vi "Load.vi"(8 "error in (no error)":errorcluster, 11 "reference in":refnum<class "DUT_Handler_Simple.lvclass">) -> (0 "error out":errorcluster, 1 "OK":bool, 3 "reference in":refnum<class "DUT_Handler_Simple.lvclass">)   [LabVIEW 2022 SP3, in "DUT_Handler_Simple.lvlib" / "DUT_Handler_Simple.lvclass"]
uses:
  DUT_Handler_Simple.lvclass
  Components/DUT_Handler_Base.lvlibp/Action.ctl
  Components/DUT_Handler_Base.lvlibp/EventData.ctl
  Components/DUT_Handler_Base.lvlibp/DUT_Handler_Base.lvclass
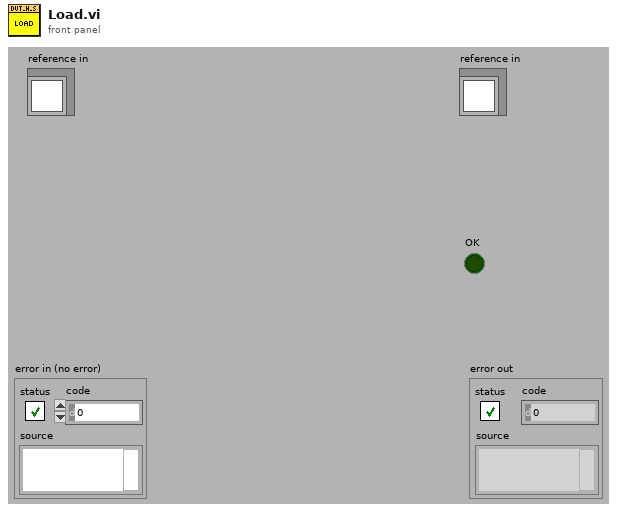
[diagram p1: front panel]
types:
  T1 = typedef "DUT_Handler_Base.lvlibp/DUT_Handler_Base.lvclass/EventData.ctl" = cluster{"Action":enum16{"Load", "Cancel", "MoveIn", "MoveOut", "Abort", "Msg", "Enabled", "Disabled", "Fault", "Shutdown"}, "SN":string, "BN":string, "DUT__ID":u32, "Message":string, "From":string, "To":string}
  T2 = typedef "DUT_Handler_Base.lvlibp/DUT_Handler_Base.lvclass/Action.ctl" = enum16{"Load", "Cancel", "MoveIn", "MoveOut", "Abort", "Msg", "Enabled", "Disabled", "Fault", "Shutdown"}
  T3 = typedef "DUT_Handler_Simple.lvlib/DUT_Handler_Simple.lvclass/ObjectAttributes.ctl" = cluster{"Config":T4, "event_data":T1, "Enabled":bool, "Barcode_Reader":refnum<class "Barcode_Reader_Base.lvclass">}
  T4 = typedef "DUT_Handler_Simple.lvlib/DUT_Handler_Simple.lvclass/Config.ctl" = cluster{"default":string}
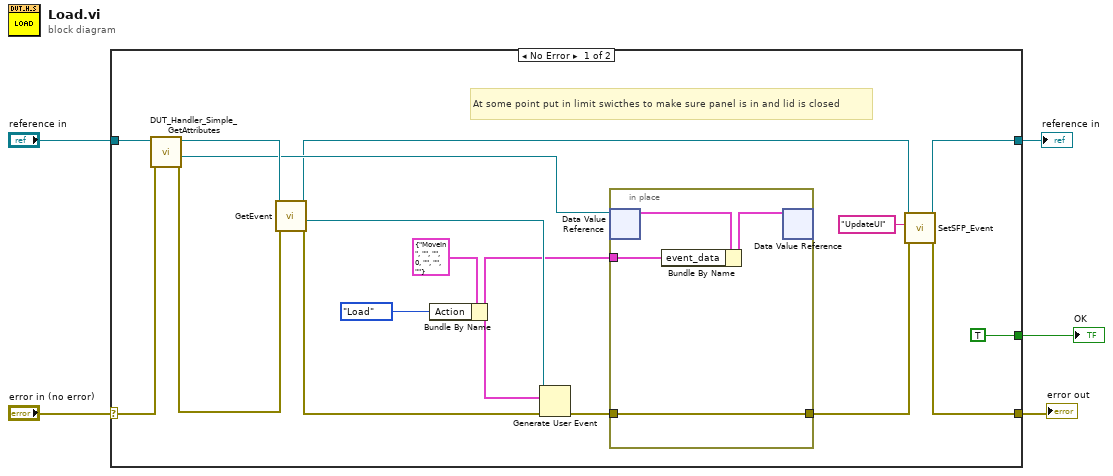
[diagram p0: block diagram]
diagram:
  n1 = case shown="No Error" "error in (no error)" {
    selector: "error in (no error)" -> [w22 w28]
    tunnel: [w7 w28] -> w4
    tunnel: [w8 w27] -> w2
    tunnel: "reference in" -> [w21 w27]
    tunnel: [TRUE _] -> w1
    frame No Error {
      # "At some point put in limit swicthes to make sure panel is in and lid is closed"
      n2 = call "DUT_Handler_Simple_GetAttributes.vi"("error in (no error)"=w22, "reference in"=w21) -> ("error out"=w18:errorcluster, "DataRef"=w14:refnum<data-value>, "reference out"=w15:refnum<class "DUT_Handler_Simple.lvclass">)  [unwired: 6 in, 1 out]
      n3 = call-dynamic "GetEvent.vi"("error in (no error)"=w18, "reference in"=w15) -> ("error out"=w17:errorcluster, "DUT_Handler"=w16:refnum<user-event>, "reference in"=w9:refnum<class "DUT_Handler_Simple.lvclass">)  [unwired: 6 in]
      n4 = Bundle By Name(cluster=T1 {"Action"=enum."MoveIn", "SN"="", "BN"="", "DUT__ID"=0, "Message"="", "From"="", "To"=""} ("event_data"), "Action"=Action."Load") -> (w13:T1)
      n5 = Generate User Event(user event=w16, event data cluster=w13, error in=w17) -> (error out=w12:errorcluster)  [unwired: 1 in, 1 out]
      n6 = in-place {
        in-place-border: w13 -> [w24]
        in-place-border: w12 -> [w23]
        in-place-border: [w23] -> w10
        n7 = in-place-dvr #1(w14) -> (w26:T3)  [unwired: 1 out]
        n8 = Bundle By Name(cluster=w26, "event_data"=w24) -> (w25:T3)
        n9 = in-place-dvr #1(w25) -> ()  [unwired: 2 out]
      }
      n10 = call-dynamic "SetSFP_Event.vi"("error in (no error)"=w10, "msg"="UpdateUI", "reference in"=w9) -> ("error out"=w7:errorcluster, "reference out"=w8:refnum<class "DUT_Handler_Simple.lvclass">)  [unwired: 7 in]
    }
    frame Error {
    }
  }
  "error out" <- w4
  "reference in" <- w2
  "OK" <- w1
